vi "Speaker ring to Left-Right ring.vi"(1 "Speaker":T2) -> (0 "Ear":T1)   [LabVIEW 2015]
doc: "Extracts \"Left\" or \"Right\" side from speaker ring."
uses:
  Speaker ring.ctl
  Left-Right ring.ctl
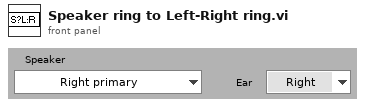
[diagram p1: front panel]
types:
  T1 = typedef "Left-Right ring.ctl" = enum16{"Right", "Left"}
  T2 = typedef "Speaker ring.ctl" = enum16{"Right primary", "Right secondary", "Left primary", "Left secondary"}
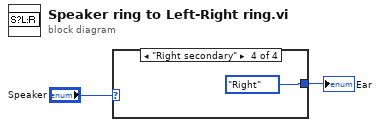
[diagram p0: block diagram]
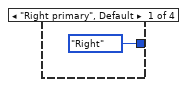
[diagram p2: hidden frame]
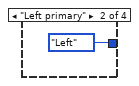
[diagram p3: hidden frame]
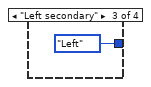
[diagram p4: hidden frame]
diagram:
  n1 = case shown="\"Right secondary\"" "Speaker" {
    tunnel: [Left-Right_ring."Right" ("Ear") Left-Right_ring."Left" ("Ear") Left-Right_ring."Left" ("Ear") Left-Right_ring."Right" ("Ear")] -> w1
    frame "Right primary", Default {
    }
    frame "Left primary" {
    }
    frame "Left secondary" {
    }
    frame "Right secondary" {
    }
  }
  "Ear" <- w1
